vi "干啮合测试.vi"(8 "error in (no error)":errorcluster caption="错误输入（无错误）") -> (0 "error out":errorcluster caption="错误输出")   [LabVIEW 2015]
doc: "该连续测量范例项目在队列消息处理器模板的基础上实现。\n\n事件处理循环负责按用户界面操作生成对应的消息。\n\n消息处理循环负责对事件处理循环或其他消息生成的消息进行处理。其中还包括用于采集和记录消息处理循环的子VI，以及用于更新图表的循环。"
uses:
  Settings/Settings.ctl
  Acquisition/Hardware Configuration.ctl
  Logging/Logging Configuration.ctl
  Motor Control/Hardware Configuration.ctl
  controls/UI Data.ctl
  controls/UI State.ctl
  Measure Type.ctl
  <vilib>/Analysis/baseanly.llb/Mean (DBL).vi
  support/Message Queue/Enqueue Message (Single).vi
  <vilib>/Utility/error.llb/Error Cluster From Error Code.vi
  <vilib>/ErrorRing/Error Ring.xnode
  Acquisition/Acquisition.lvlib
  Logging/Logging.lvlib
  Settings/Settings.lvlib
  support/User Event - Stop/User Event - Stop.lvlib
  support/Message Queue/Message Queue.lvlib
  Motor Control/Motor Control.lvlib
  <vilib>/Analysis/NI_AALBase.lvlib
panel:
  out "XY Graph":cluster{"Y":dbl[], "Y":dbl[]}[](graph) caption="角度VS扭矩图"
  in  "设置":bool
  in  "清零":bool
  in  "读取":bool
  out "模拟通道5":dbl
  out "流量":dbl
  out "右推力":dbl
  out "左推力":dbl
  out "油压":dbl
  out "扭矩":dbl
  out "角度":dbl
  in  "计算":bool
  in  "Start":bool caption="开始"
  in  "Stop":bool caption="停止"
  out "Status":string caption="状态"
  in  "Exit":bool caption="退出"
  # "干啮合测试"
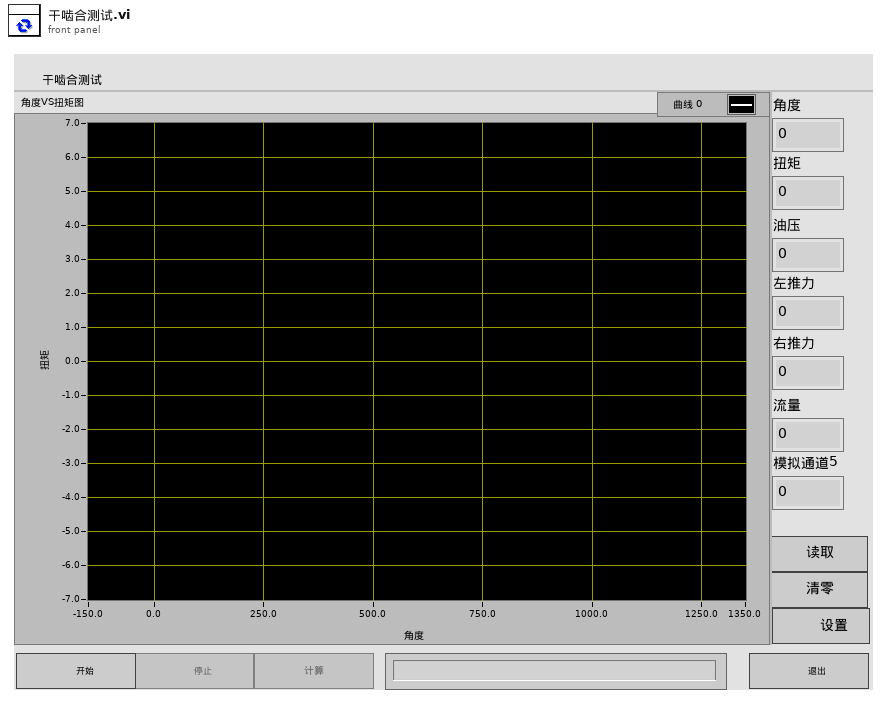
[diagram p1: front panel]
types:
  T1 = typedef "Motor Control.lvlib/电机转动逻辑1.ctl" = cluster{"反转判断条件1":T2, "停止判断条件1":T3}
  T2 = typedef "Motor Control.lvlib/反转判断条件1.ctl" = cluster{"传感器序号":i32, "条件":enum16{"小于", "大于", "等于"}, "值":dbl, "条件判断时间间隔":i32}
  T3 = typedef "Motor Control.lvlib/停止判断条件1.ctl" = cluster{"角度传感器序号":i32, "正转/反转":enum16{"正转", "反转"}, "反转次数":i32, "停止角度":dbl, "停止角度误差范围":dbl}
  T4 = typedef "UI State.ctl" = enum16{"Idle", "Acquiring and Logging", "Waiting for Exit", "Waiting for Exit (Acq Stopped)", "Waiting for Exit (Log Stopped)", "Waiting for Stop", "Waiting for Stop (Acq Stopped)", "Waiting for Stop (Log Stopped)"}
  T5 = typedef "UI Data.ctl" = cluster{"Start Ref":refnum<vi>, "Stop Ref":refnum<vi>, "calculate Ref":refnum<vi>, "Status Ref":refnum<vi>, "Exit Ref":refnum<vi>, "read Ref":refnum<vi>, "clean Ref":refnum<vi>}
  T6 = typedef "Settings.lvlib/Settings.ctl" = cluster{"Hardware Configuration":T7, "Logging Configuration":T8, "电机设置":T9, "啮合测试电机转动逻辑":T1, "功能测试电机转动逻辑":T1, "力提特性电机转动逻辑":T1}
  T7 = typedef "Acquisition.lvlib/Hardware Configuration.ctl" = cluster{"电压读取设置":cluster{"DAQmx Channel":tag, "Max Input":dbl, "Min Input":dbl, "Sample Rate":dbl, "Sample Number":i32, "DAQmx Task":refnum<k21>, "device in":tag}, "角度传感器设置":cluster{"counter":tag, "units":i32, "分辨率":i32, "初始角度":dbl, "DecodingType":i32, "A相端口":tag, "B相端口":tag, "task in":refnum<k21>}}
  T8 = typedef "Logging.lvlib/Logging Configuration.ctl" = cluster{"Log File Base Path":path, "电压传感器转换率":dbl[], "电压传感器本底":dbl[]}
  T9 = typedef "Motor Control.lvlib/Hardware Configuration.ctl" = cluster{"counter":tag, "方向端口":tag, "当前方向":bool, "频率":dbl, "DAQmx Task":refnum<k21>}
  T10 = typedef "Message Queue.lvlib/All Message Queues.ctl" = cluster{"UI":refnum<queue>, "Acquisition":refnum<queue>, "Logging":refnum<queue>, "MotorCtrl":refnum<queue>, "plot logic":refnum<queue>}
  T11 = typedef "Measure Type.ctl" = enum16{"啮合", "退回", "功能", "力特性"}
  T12 = enum8{"Enabled", "Disabled", "Disabled and Grayed Out"}
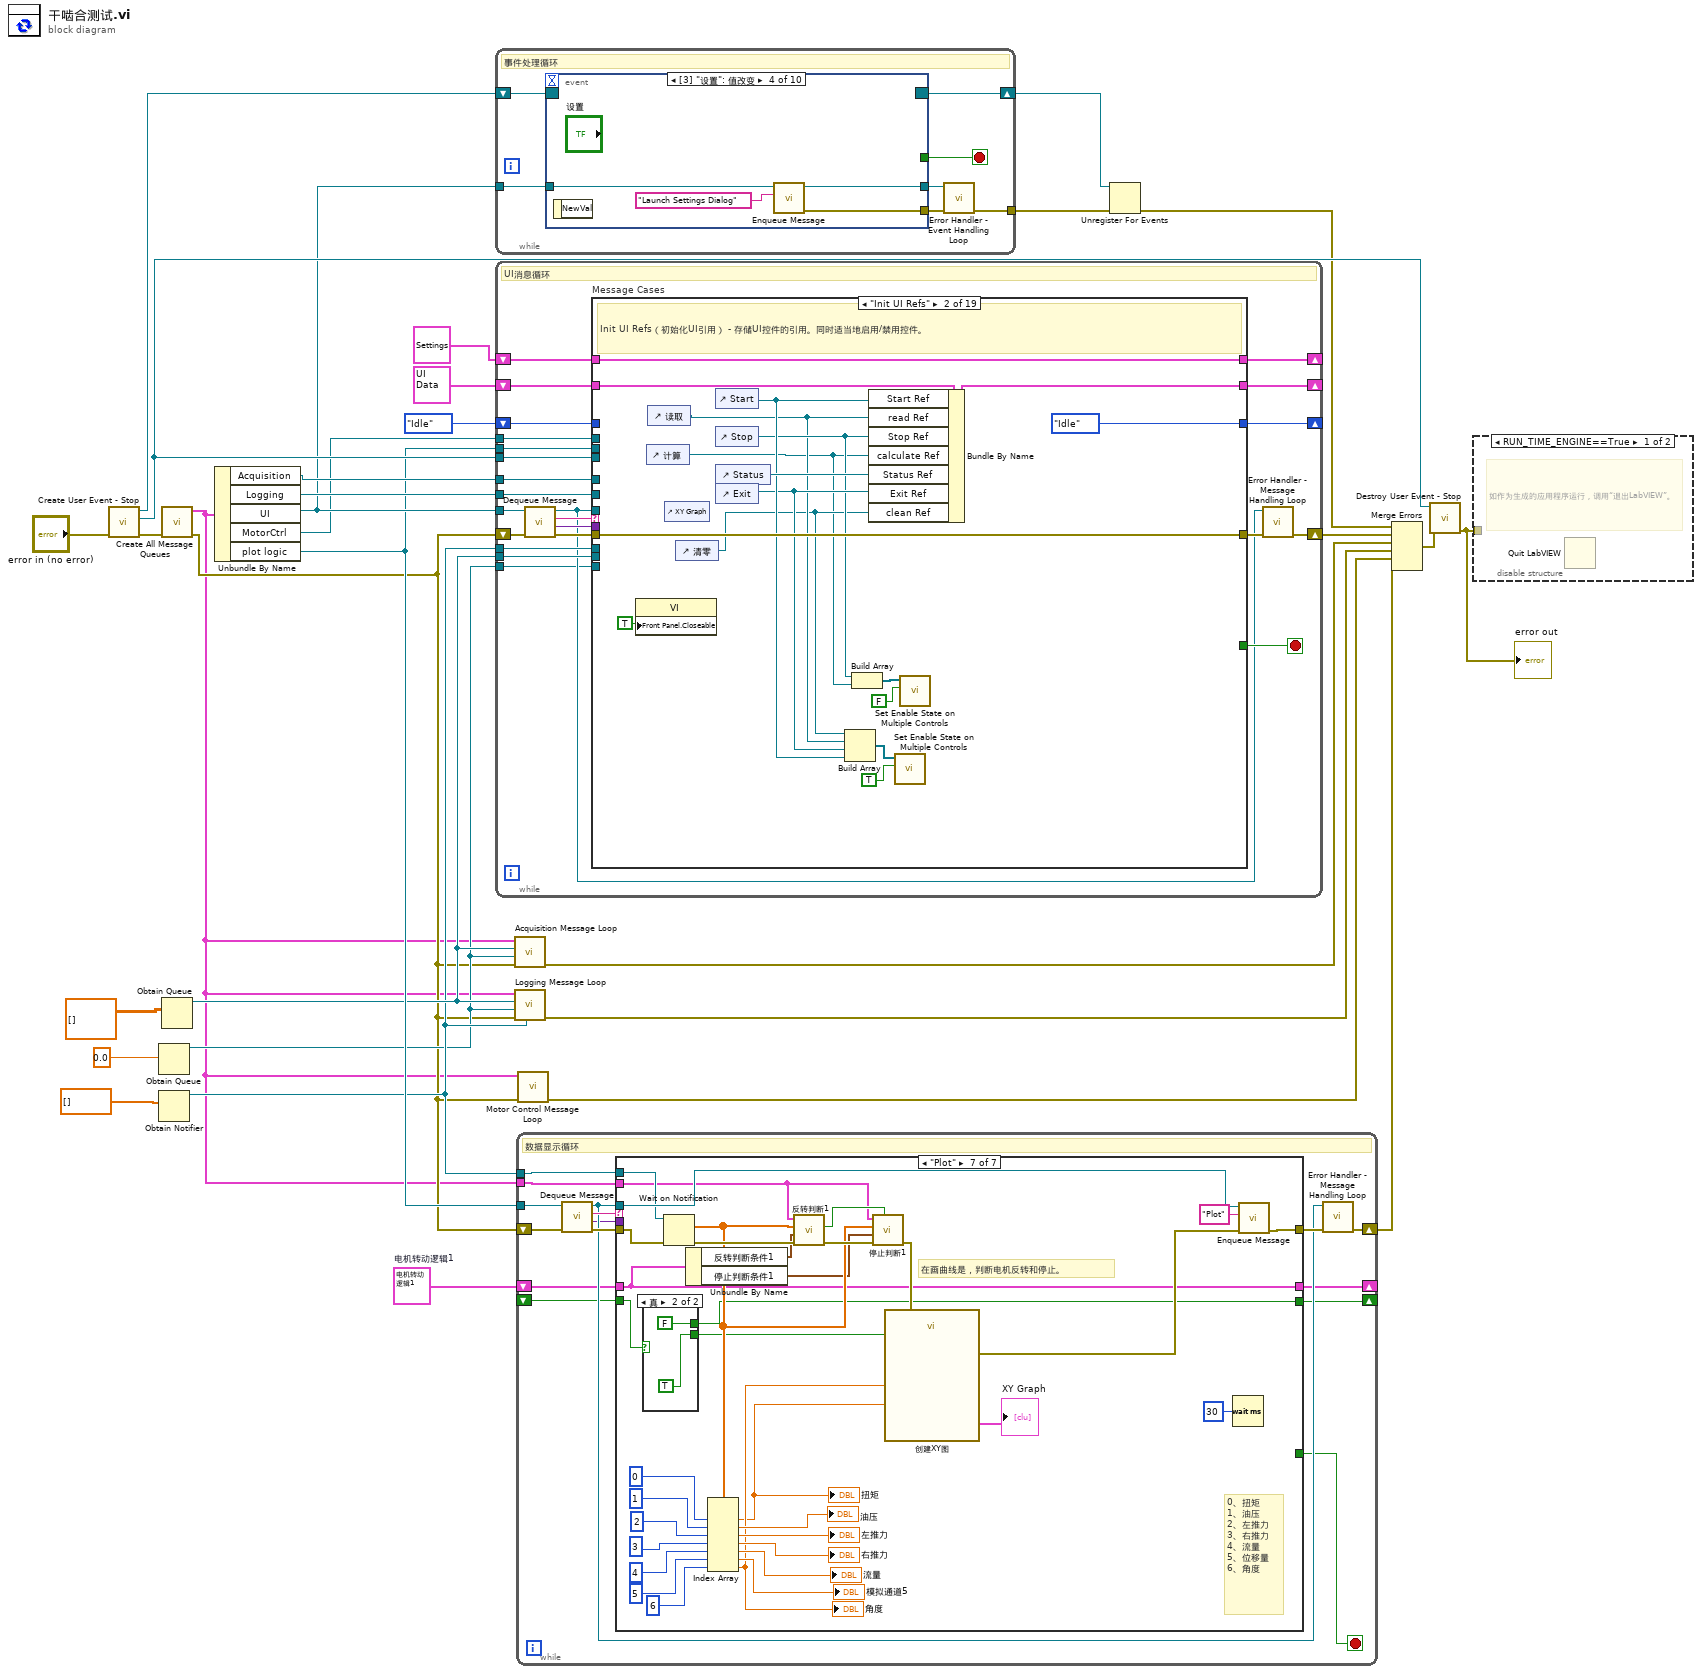
[diagram p0: block diagram]
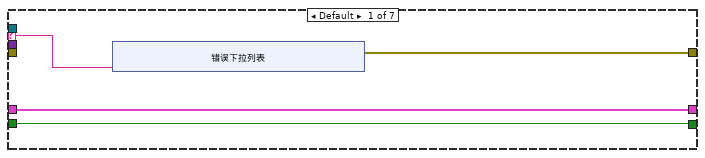
[diagram p3: hidden frame]
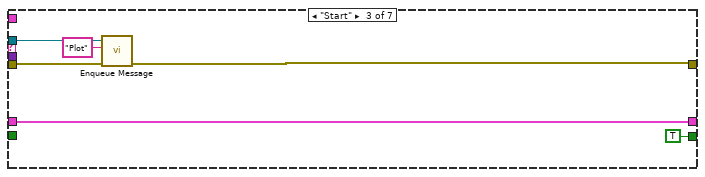
[diagram p5: hidden frame]
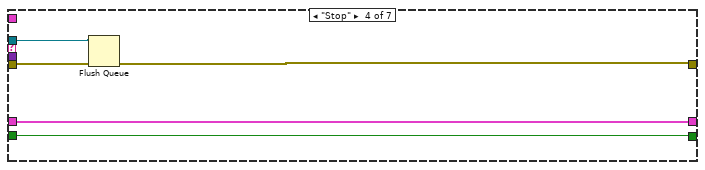
[diagram p6: hidden frame]
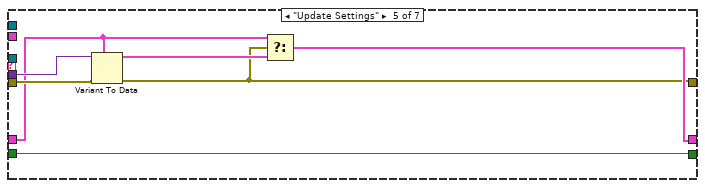
[diagram p7: hidden frame]
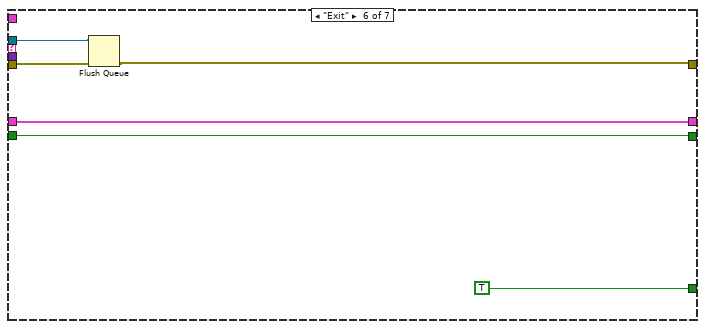
[diagram p8: hidden frame]
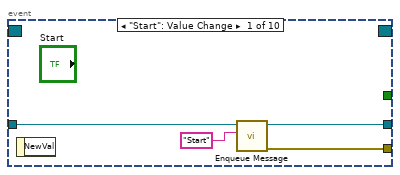
[diagram p10: hidden frame]
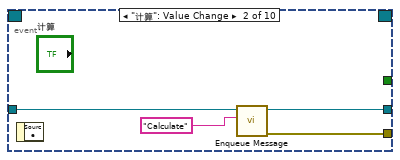
[diagram p11: hidden frame]
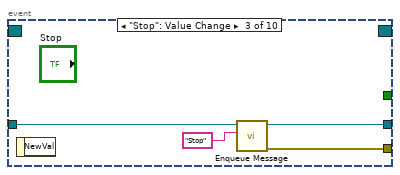
[diagram p12: hidden frame]
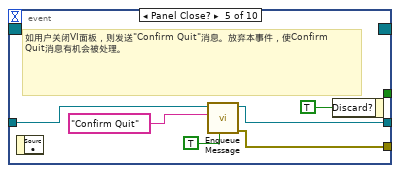
[diagram p13: hidden frame]
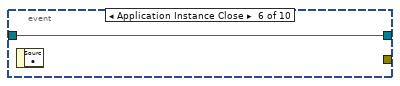
[diagram p14: hidden frame]
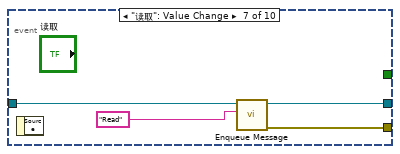
[diagram p15: hidden frame]
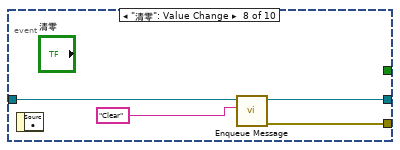
[diagram p16: hidden frame]
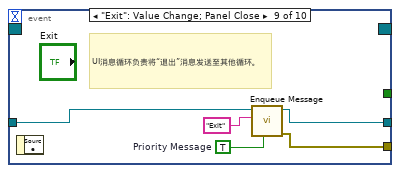
[diagram p17: hidden frame]
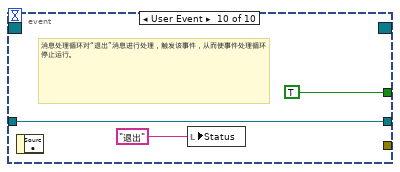
[diagram p18: hidden frame]
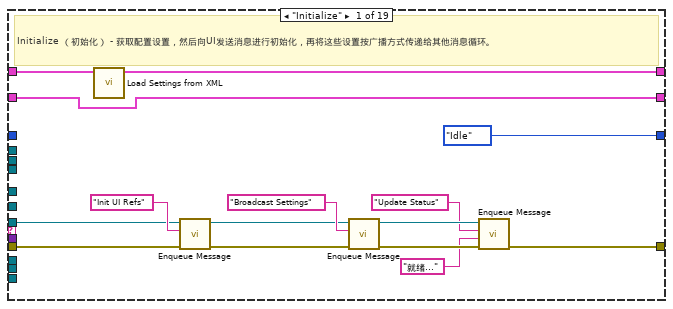
[diagram p19: hidden frame]
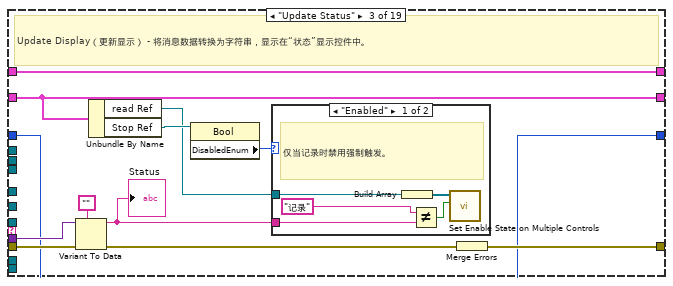
[diagram p20: hidden frame]
diagram:
  w3 = T1 {"反转判断条件1"={"传感器序号"=0, "条件"=enum."小于", "值"=0.0, "条件判断时间间隔"=0}, "停止判断条件1"={"角度传感器序号"=0, "正转/反转"=enum."正转", "反转次数"=0, "停止角度"=0.0, "停止角度误差范围"=0.0}}  # 电机转动逻辑1
  n1 = call "Create User Event - Stop.vi"("error in (no error)"="error in (no error)") -> ("error out"=w25:errorcluster, "User Event - Stop"=w27:refnum<user-event>, "Stop Event Registration Refnum"=w28:refnum<event-registration>)  [unwired: 8 in]
  n2 = Obtain Queue(element data type=0.0) -> (queue out=w8:refnum<queue>)  [unwired: 4 in, 2 out]
  n3 = Obtain Notifier(notification data type=dbl[] []) -> (notifier out=w10:refnum<notifier>)  [unwired: 3 in, 2 out]
  n4 = call "Create All Message Queues.vi"("error in (no error)"=w25) -> ("error out"=w7:errorcluster, "Message Queues out"=w4:T10)  [unwired: 9 in]
  n5 = Obtain Queue(element data type=dbl[][] []) -> (queue out=w11:refnum<queue>)  [unwired: 4 in, 2 out]
  n6 = Unbundle By Name(w4) -> ("Acquisition"=w19:refnum<queue>, "Logging"=w18:refnum<queue>, "UI"=w17:refnum<queue>, "MotorCtrl"=w15:refnum<queue>, "plot logic"=w14:refnum<queue>)
  n7 = while {
    tunnel: w17 -> [w37]
    tunnel: [w32] -> w30
    shift-right: [w36] -> w21
    shift-left: w28 -> [w38]
    stop <- w35 stop-if-true
    # "事件处理循环"
    n8 = event shown="[3] \"设置\": 值改变" {
      selector: w38 -> [_ _ _ _ _ _ _ _ _ _]
      dyn-events: [_ _ _ _ _ _ _ _ _ _] -> w36
      timeout: _ -> [_ _ _ _ _ _ _ _ _ _]
      tunnel: [_ _ _ _ _ _ _ _ _ TRUE ("Discard?")] -> w35
      tunnel: w37 -> [w40 w45 w49 w53 w60 w61 w63 w67 w71 w75]
      tunnel: [w42 w44 w48 w52 w55 _ w65 w69 w74 _] -> w33
      tunnel: [w39 w43 w47 w51 w56 w61 w62 w66 w70 w75] -> w34
      event "Start": Value Change {
        n9 = event-data() -> ()  [unwired: 1 in, 1 out]
        n10 = call-poly "Enqueue Message.vi"("Message"="Start", "Message Queue"=w40) -> ("error out"=w42:errorcluster, "dup Message Queue"=w39:refnum<queue>)  [unwired: 8 in]
      }
      event "计算": Value Change {
        n11 = event-data() -> ()  [unwired: 1 in, 1 out]
        n12 = call-poly "Enqueue Message.vi"("Message"="Calculate", "Message Queue"=w45) -> ("error out"=w44:errorcluster, "dup Message Queue"=w43:refnum<queue>)  [unwired: 8 in]
      }
      event "Stop": Value Change {
        n13 = event-data() -> ()  [unwired: 1 in, 1 out]
        n14 = call-poly "Enqueue Message.vi"("Message"="Stop", "Message Queue"=w49) -> ("error out"=w48:errorcluster, "dup Message Queue"=w47:refnum<queue>)  [unwired: 8 in]
      }
      event "设置": Value Change {
        n15 = event-data() -> ()  [unwired: 1 in, 1 out]
        n16 = call-poly "Enqueue Message.vi"("Message"="Launch Settings Dialog", "Message Queue"=w53) -> ("error out"=w52:errorcluster, "dup Message Queue"=w51:refnum<queue>)  [unwired: 8 in]
      }
      event Panel Close? {
        # "如用户关闭VI面板，则发送\"Confirm Quit\"消息。放弃本事件，使Confirm Quit消息有机会被处理。"
        n17 = event-data() -> ()  [unwired: 1 in, 1 out]
        n18 = call-poly "Enqueue Message.vi"("Priority Message? (F)"=TRUE, "Message"="Confirm Quit", "Message Queue"=w60) -> ("error out"=w55:errorcluster, "dup Message Queue"=w56:refnum<queue>)  [unwired: 7 in]
        n19 = event-data("Discard?"=TRUE) -> ()  [unwired: 1 in, 1 out]
      }
      event Application Instance Close {
        n20 = event-data() -> ()  [unwired: 1 in, 1 out]
      }
      event "读取": Value Change {
        n21 = event-data() -> ()  [unwired: 1 in, 1 out]
        n22 = call-poly "Enqueue Message.vi"("Message"="Read", "Message Queue"=w63) -> ("error out"=w65:errorcluster, "dup Message Queue"=w62:refnum<queue>)  [unwired: 8 in]
      }
      event "清零": Value Change {
        n23 = event-data() -> ()  [unwired: 1 in, 1 out]
        n24 = call-poly "Enqueue Message.vi"("Message"="Clear", "Message Queue"=w67) -> ("error out"=w69:errorcluster, "dup Message Queue"=w66:refnum<queue>)  [unwired: 8 in]
      }
      event "Exit": Value Change; Panel Close {
        w72 = TRUE  # Priority Message
        # "UI消息循环负责将“退出”消息发送至其他循环。"
        n25 = event-data() -> ()  [unwired: 1 in, 1 out]
        n26 = call-poly "Enqueue Message.vi"("Priority Message? (F)"=w72, "Message"="Exit", "Message Queue"=w71) -> ("error out"=w74:errorcluster, "dup Message Queue"=w70:refnum<queue>)  [unwired: 7 in]
      }
      event User Event {
        # "消息处理循环对“退出”消息进行处理，触发该事件，从而使事件处理循环停止运行。"
        n27 = event-data() -> ()  [unwired: 1 in, 1 out]
        n28 = local write "Status"("退出" ("Exit String")) -> ()
      }
    }
    n29 = call "Error Handler - Event Handling Loop.vi"("error in (no error)"=w33, "Message Queue"=w34) -> ("dup error in"=w32:errorcluster)  [unwired: 8 in, 1 out]
  }
  n30 = while {
    tunnel: w17 -> [w94]
    tunnel: w27 -> [w99]
    shift-right: [w84] -> w31
    shift-left: w7 -> [w98]
    shift-right: [w93] -> _
    shift-left: T6 {"Hardware Configuration"={"电压读取设置"={"DAQmx Channel"="", "Max Input"=0.0, "Min Input"=0.0, "Sample Rate"=0.0, "Sample Number"=0, "DAQmx Task"="", "device in"=""}, "角度传感器设置"={"counter"="Dev1/ctr0", "units"=10146, "分辨率"=0, "初始角度"=0.0, "DecodingType"=10092, "A相端口"="/Dev1/PFI8", "B相端口"="/Dev1/PFI8", "task in"=""}}, "Logging Configuration"={"Log File Base Path"=path "", "电压传感器转换率"=[], "电压传感器本底"=[]}, "电机设置"={"counter"="Dev1/ctr0", "方向端口"="", "当前方向"=FALSE, "频率"=0.0, "DAQmx Task"=""}, "啮合测试电机转动逻辑"={"反转判断条件1"={"传感器序号"=0, "条件"=enum."小于", "值"=0.0, "条件判断时间间隔"=0}, "停止判断条件1"={"角度传感器序号"=0, "正转/反转"=enum."正转", "反转次数"=0, "停止角度"=0.0, "停止角度误差范围"=0.0}}, "功能测试电机转动逻辑"={"反转判断条件1"={"传感器序号"=0, "条件"=enum."小于", "值"=0.0, "条件判断时间间隔"=0}, "停止判断条件1"={"角度传感器序号"=0, "正转/反转"=enum."正转", "反转次数"=0, "停止角度"=0.0, "停止角度误差范围"=0.0}}, "力提特性电机转动逻辑"={"反转判断条件1"={"传感器序号"=0, "条件"=enum."小于", "值"=0.0, "条件判断时间间隔"=0}, "停止判断条件1"={"角度传感器序号"=0, "正转/反转"=enum."正转", "反转次数"=0, "停止角度"=0.0, "停止角度误差范围"=0.0}}} ("Settings") -> [w92]
    shift-right: [w90] -> _
    shift-left: T5 {"Start Ref"=refnum, "Stop Ref"=refnum, "calculate Ref"=refnum, "Status Ref"=refnum, "Exit Ref"=refnum, "read Ref"=refnum, "clean Ref"=refnum} ("Measurement UI Controls") -> [w91]
    tunnel: w19 -> [w89]
    tunnel: w18 -> [w88]
    tunnel: w10 -> [w87]
    tunnel: w11 -> [w86]
    shift-right: [w81] -> _
    shift-left: UI_State."Idle" ("UI State") -> [w82]
    tunnel: w15 -> [w78]
    tunnel: w14 -> [w79]
    tunnel: w8 -> [w80]
    stop <- w100 stop-if-true
    # "UI消息循环"
    n31 = call "Dequeue Message.vi"("error in (no error)"=w98, "Message Queue"=w94) -> ("error out"=w97:errorcluster, "Message Data"=w95:variant, "Message"=w96:string, "dup Message Queue"=w83:refnum<queue>)  [unwired: 6 in]
    n32 = case "Message Cases" shown="\"Init UI Refs\"" w96 {
      selector: w96 -> [_ _ _ _ _ _ _ _ _ _ _ _ _ _ _ _ _ _ w430]
      tunnel: w83 -> [w105 _ _ w179 _ w219 w223 w248 _ w296 w317 w323 w361 _ _ w389 _ _ _]
      tunnel: w97 -> [w104 w132 w143 w178 w185 w218 w225 w250 w273 w298 w310 w322 w368 w375 w379 w392 w416 w424 _]
      tunnel: [w111 w132 w144 w180 w188 w220 w224 w249 w290 w293 w313 w321 w369 w374 w382 w395 w419 w428 w431] -> w85
      tunnel: [_ _ _ _ _ _ _ _ _ _ _ _ TRUE _ _ _ _ _ _] -> w100
      tunnel: w95 -> [_ _ w142 _ _ _ _ _ _ _ w309 _ _ _ _ _ _ _ _]
      tunnel: w99 -> [_ _ _ _ _ _ _ _ _ _ _ _ w367 _ _ _ _ _ _]
      tunnel: [w114 w131 w139 w177 w187 w217 w229 w254 w288 w295 w319 w326 w365 w373 w377 w385 w401 w427 w433] -> w93
      tunnel: w92 -> [w115 w131 w139 w177 w187 w217 w229 w254 w288 w299 w319 w326 w365 w373 w377 w386 w401 w427 w433]
      tunnel: w91 -> [w107 w130 w138 w174 w186 w214 w228 w253 w285 w292 w318 w325 w364 w372 w381 w394 w418 w426 w432]
      tunnel: [w107 w129 w138 w174 w186 w214 w228 w253 w285 w292 w318 w325 w364 w372 w381 w394 w418 w426 w432] -> w90
      tunnel: w89 -> [_ _ _ w162 _ w202 _ _ w284 _ _ _ w363 _ _ _ _ _ _]
      tunnel: w88 -> [_ _ _ w164 w182 w205 _ _ w283 _ _ _ w362 _ _ _ _ w422 _]
      tunnel: w87 -> [_ _ _ _ _ _ _ _ _ _ _ _ w360 _ _ _ _ _ _]
      tunnel: w86 -> [_ _ _ _ _ _ _ _ _ _ _ _ w357 _ _ _ _ _ _]
      tunnel: w82 -> [_ _ w133 _ w181 w200 w227 w252 w282 w291 w312 w324 _ w371 w380 w393 w417 w425 w429]
      tunnel: [UI_State."Idle" ("UI State") UI_State."Idle" ("UI State") w133 UI_State."Acquiring and Logging" ("UI State") w181 w199 w226 w251 w282 w291 w312 w320 UI_State."Idle" ("UI State") w371 w380 w393 w417 w425 w429] -> w81
      tunnel: w80 -> [_ _ _ _ _ _ _ _ _ _ _ _ w352 _ _ _ _ _ _]
      tunnel: w79 -> [_ _ _ w156 _ w192 _ _ w277 _ _ _ w351 _ _ _ _ _ _]
      tunnel: w78 -> [_ _ _ w152 _ w190 _ _ w280 _ _ _ w350 _ _ _ _ _ _]
      frame "Initialize" {
        # "Initialize （初始化） - 获取配置设置，然后向UI发送消息进行初始化，再将这些设置按广播方式传递给其他消息循环。"
        n33 = call "Load Settings from XML.vi"("Settings in"=w115) -> ("Settings out"=w114:T6)  [unwired: 9 in, 1 out]
        n34 = call-poly "Enqueue Message.vi"("error in (no error)"=w104, "Message"="Init UI Refs", "Message Queue"=w105) -> ("error out"=w102:errorcluster, "dup Message Queue"=w103:refnum<queue>)  [unwired: 7 in]
        n35 = call-poly "Enqueue Message.vi"("error in (no error)"=w102, "Message"="Broadcast Settings", "Message Queue"=w103) -> ("error out"=w113:errorcluster, "dup Message Queue"=w112:refnum<queue>)  [unwired: 7 in]
        n36 = call-poly "Enqueue Message.vi"("error in (no error)"=w113, "Message Data"="就绪..." ("Ready..."), "Message"="Update Status", "Message Queue"=w112) -> ("error out"=w111:errorcluster)  [unwired: 6 in, 1 out]
      }
      frame "Init UI Refs" {
        # "Init UI Refs（初始化UI引用） - 存储UI控件的引用。同时适当地启用/禁用控件。"
        n37 = property class="VI"("Front Panel.Closeable"=TRUE ("Front Panel Window:Closeable")) -> ()  [unwired: 2 in, 2 out]
        n38 = control-ref of="计算"() -> (w116:refnum<vi>)
        n39 = control-ref of="读取"() -> (w118:refnum<vi>)
        n40 = control-ref of="XY Graph"() -> ()  [unwired: 1 out]
        n41 = control-ref of="清零"() -> (w117:refnum<vi>)
        n42 = control-ref of="Start"() -> (w125:refnum<vi>)
        n43 = control-ref of="Stop"() -> (w121:refnum<vi>)
        n44 = control-ref of="Status"() -> (w126:refnum<vi>)
        n45 = control-ref of="Exit"() -> (w122:refnum<vi>)
        n46 = Build Array(w117, w118, w122, w125) -> (w124:refnum<vi>[])
        n47 = Build Array(w121, w116) -> (w120:refnum<vi>[])
        n48 = Bundle By Name(cluster=w130, "Start Ref"=w125, "read Ref"=w118, "Stop Ref"=w121, "calculate Ref"=w116, "Status Ref"=w126, "Exit Ref"=w122, "clean Ref"=w117) -> (w129:T5)
        n49 = call "Set Enable State on Multiple Controls.vi"("Enable?"=TRUE, "Controls"=w124) -> ()  [unwired: 10 in]
        n50 = call "Set Enable State on Multiple Controls.vi"("Enable?"=FALSE, "Controls"=w120) -> ()  [unwired: 10 in]
      }
      frame "Update Status" {
        # "Update Display（更新显示） - 将消息数据转换为字符串，显示在“状态”显示控件中。"
        n51 = Variant To Data(error in=w143, type="", Variant=w142) -> (data=w135:string, error out=w140:errorcluster)
        "Status" <- w135
        n52 = Unbundle By Name(w138) -> ("read Ref"=w134:refnum<vi>, "Stop Ref"=w137:refnum<vi>)
        n53 = property class="Bool"(reference=w137) -> ("DisabledEnum"=w136:T12)  [unwired: 1 in, 2 out]
        n54 = case shown="\"Enabled\"" w136 {
          tunnel: w135 -> [w147 _]
          tunnel: w134 -> [w148 _]
          frame "Enabled" {
            # "仅当记录时禁用强制触发。"
            n55 = Build Array(w148) -> (w149:refnum<vi>[])
            n56 = Not Equal?(x="记录" ("Logging"), y=w147) -> (x != y?=w145:bool)
            n57 = call "Set Enable State on Multiple Controls.vi"("Enable?"=w145, "Controls"=w149) -> ()  [unwired: 10 in]
          }
          frame "Disabled", Default {
          }
        }
        n58 = Merge Errors(w140) -> (w144:errorcluster)
      }
      frame "Start" {
        # "启用：停止\n禁用：开始、退出、设置"
        # "Start（开始） - 对于已经开始的采集，启用/禁用各个按钮并更新状态显示。"
        n59 = Unbundle By Name(w174) -> ("Stop Ref"=w157:refnum<vi>, "clean Ref"=w158:refnum<vi>, "read Ref"=w159:refnum<vi>, "Start Ref"=w169:refnum<vi>, "Exit Ref"=w168:refnum<vi>, "calculate Ref"=w167:refnum<vi>)
        n60 = call-poly "Enqueue Message.vi"("error in (no error)"=w178, "Message Data"="开始" ("Waiting for trigger"), "Message"="Update Status", "Message Queue"=w179) -> ("error out"=w166:errorcluster)  [unwired: 6 in, 1 out]
        n61 = Build Array(w157) -> (w171:refnum<vi>[])
        n62 = Build Array(w158, w159, w169, w168, w167) -> (w172:refnum<vi>[])
        n63 = call-poly "Enqueue Message.vi"("error in (no error)"=w166, "Message"="Start", "Message Queue"=w164) -> ("error out"=w163:errorcluster)  [unwired: 7 in, 1 out]
        n64 = call "Set Enable State on Multiple Controls.vi"("Enable?"=TRUE, "Controls"=w171) -> ()  [unwired: 10 in]
        n65 = call "Set Enable State on Multiple Controls.vi"("Enable?"=FALSE, "Controls"=w172) -> ()  [unwired: 10 in]
        n66 = call-poly "Enqueue Message.vi"("error in (no error)"=w163, "Message"="Start", "Message Queue"=w162) -> ("error out"=w154:errorcluster)  [unwired: 7 in, 1 out]
        n67 = call-poly "Enqueue Message.vi"("error in (no error)"=w154, "Message"="Start", "Message Queue"=w156) -> ("error out"=w153:errorcluster)  [unwired: 7 in, 1 out]
        n68 = call-poly "Enqueue Message.vi"("error in (no error)"=w153, "Message"="Start", "Message Queue"=w152) -> ("error out"=w150:errorcluster)  [unwired: 7 in, 1 out]
        n69 = Merge Errors(w150) -> (w180:errorcluster)
      }
      frame "Force Trigger" {
        # "Force Trigger（强制触发） - 发送消息至记录消息循环，开始记录。"
        n70 = call-poly "Enqueue Message.vi"("error in (no error)"=w185, "Message"="Force Trigger", "Message Queue"=w182) -> ("error out"=w184:errorcluster)  [unwired: 7 in, 1 out]
        n71 = Merge Errors(w184) -> (w188:errorcluster)
      }
      frame "Stop" {
        # "停止画图、电机、记录，最后停止采集。"
        # "启用：开始、退出、设置\n禁用：停止"
        # "停止－对于已经停止的采集，启用/禁用各个按钮并更新状态显示。"
        n72 = Unbundle By Name(w214) -> ("Stop Ref"=w196:refnum<vi>, "read Ref"=w197:refnum<vi>, "clean Ref"=w198:refnum<vi>, "Start Ref"=w209:refnum<vi>, "Exit Ref"=w208:refnum<vi>, "calculate Ref"=w207:refnum<vi>)
        n73 = call-poly "Enqueue Message.vi"("error in (no error)"=w218, "Message Data"="就绪..." ("Ready..."), "Message"="Update Status", "Message Queue"=w219) -> ("error out"=w195:errorcluster)  [unwired: 6 in, 1 out]
        n74 = Build Array(w197, w198, w209, w208, w207) -> (w212:refnum<vi>[])
        n75 = Build Array(w196) -> (w211:refnum<vi>[])
        n76 = call "Set Enable State on Multiple Controls.vi"("Enable?"=TRUE, "Controls"=w212) -> ()  [unwired: 10 in]
        n77 = call "Set Enable State on Multiple Controls.vi"("Enable?"=FALSE, "Controls"=w211) -> ()  [unwired: 10 in]
        n78 = call-poly "Enqueue Message.vi"("error in (no error)"=w195, "Message"="Stop", "Message Queue"=w192) -> ("error out"=w194:errorcluster)  [unwired: 7 in, 1 out]
        n79 = call-poly "Enqueue Message.vi"("error in (no error)"=w194, "Message"="Stop", "Message Queue"=w190) -> ("error out"=w193:errorcluster)  [unwired: 7 in, 1 out]
        n80 = call-poly "Enqueue Message.vi"("error in (no error)"=w193, "Message"="Stop", "Message Queue"=w205) -> ("error out"=w204:errorcluster)  [unwired: 7 in, 1 out]
        n81 = case shown="默认" w200 {
          selector: w200 -> [_ w222]
          tunnel: [UI_State."Waiting for Stop" ("UI State") w222] -> w199
          frame Default {
          }
          frame "Waiting for Exit" {
          }
        }
        n82 = call-poly "Enqueue Message.vi"("error in (no error)"=w204, "Message"="Stop", "Message Queue"=w202) -> ("error out"=w203:errorcluster)  [unwired: 7 in, 1 out]
        n83 = Merge Errors(w203) -> (w220:errorcluster)
      }
      frame "Acquisition Stopped" {
        # "此处代码用于确定采集停止时采取何种操作。"
        n84 = case shown="\"Waiting for Stop (Log Stopped)\"" w227 {
          selector: w227 -> [w231 _ _ _ _]
          tunnel: [w231 UI_State."Waiting for Exit (Acq Stopped)" ("UI State") UI_State."Waiting for Stop (Acq Stopped)" ("UI State") UI_State."Idle" ("UI State") UI_State."Idle" ("UI State")] -> w226
          tunnel: w225 -> [w230 w232 w234 w240 w246]
          tunnel: [w230 w232 w234 w239 w245] -> w224
          tunnel: w223 -> [_ _ _ w238 w244]
          frame Default {
          }
          frame "Waiting for Exit", "Waiting for Exit (Acq Stopped)" {
          }
          frame "Waiting for Stop", "Waiting for Stop (Acq Stopped)" {
          }
          frame "Waiting for Exit (Log Stopped)" {
            # "如果正在等待退出且记录已结束，“采集停止”消息表示应退出。"
            n85 = call-poly "Enqueue Message.vi"("Priority Message? (F)"=TRUE, "error in (no error)"=w240, "Message"="Exit", "Message Queue"=w238) -> ("error out"=w239:errorcluster)  [unwired: 6 in, 1 out]
          }
          frame "Waiting for Stop (Log Stopped)" {
            # "当前状态为等待停止时，如已停止记录，则收到\"Acquisition Stopped\"消息时即可停止。"
            n86 = call-poly "Enqueue Message.vi"("error in (no error)"=w246, "Message Data"="Ready..." ("Message"), "Message"="Update Status", "Message Queue"=w244) -> ("error out"=w245:errorcluster)  [unwired: 6 in, 1 out]
          }
        }
      }
      frame "Logging Stopped" {
        # "此处代码用于确定记录停止时采取何种操作。"
        n87 = case shown="\"Waiting for Stop (Acq Stopped)\"" w252 {
          selector: w252 -> [w256 _ _ _ _]
          tunnel: [w256 UI_State."Waiting for Exit (Log Stopped)" ("UI State") UI_State."Waiting for Stop (Log Stopped)" ("UI State") UI_State."Idle" ("UI State") UI_State."Idle" ("UI State")] -> w251
          tunnel: w250 -> [w255 w257 w259 w265 w271]
          tunnel: [w255 w257 w259 w264 w270] -> w249
          tunnel: w248 -> [_ _ _ w263 w269]
          frame Default {
          }
          frame "Waiting for Exit", "Waiting for Exit (Log Stopped)" {
          }
          frame "Waiting for Stop", "Waiting for Stop (Log Stopped)" {
          }
          frame "Waiting for Exit (Acq Stopped)" {
            # "如果正在等待退出且采集已结束，“记录停止”消息表示应退出。"
            n88 = call-poly "Enqueue Message.vi"("Priority Message? (F)"=TRUE, "error in (no error)"=w265, "Message"="Exit", "Message Queue"=w263) -> ("error out"=w264:errorcluster)  [unwired: 6 in, 1 out]
          }
          frame "Waiting for Stop (Acq Stopped)" {
            # "如果正在等待停止且采集已结束，“记录停止”消息表示应停止。"
            n89 = call-poly "Enqueue Message.vi"("error in (no error)"=w271, "Message Data"="Ready..." ("Message"), "Message"="Update Status", "Message Queue"=w269) -> ("error out"=w270:errorcluster)  [unwired: 6 in, 1 out]
          }
        }
      }
      frame "Broadcast settings" {
        w276 = "Update Settings" ("Message")
        # "向“记录和采集”消息队列发送“更新设置”消息。"
        n90 = Unbundle By Name(w288) -> ("Hardware Configuration"=w287:T7, "Logging Configuration"=w286:T8, "电机设置"=w279:T9, "啮合测试电机转动逻辑"=w275:T1)
        n91 = call-poly "Enqueue Message.vi"("error in (no error)"=w273, "Message Data"=w287, "Message"=w276, "Message Queue"=w284) -> ("error out"=w289:errorcluster)  [unwired: 6 in, 1 out]
        n92 = call-poly "Enqueue Message.vi"("error in (no error)"=w289, "Message Data"=w286, "Message"=w276, "Message Queue"=w283) -> ("error out"=w281:errorcluster)  [unwired: 6 in, 1 out]
        n93 = call-poly "Enqueue Message.vi"("error in (no error)"=w281, "Message Data"=w279, "Message"=w276, "Message Queue"=w280) -> ("error out"=w278:errorcluster)  [unwired: 6 in, 1 out]
        n94 = call-poly "Enqueue Message.vi"("error in (no error)"=w278, "Message Data"=w275, "Message"=w276, "Message Queue"=w277) -> ("error out"=w274:errorcluster)  [unwired: 6 in, 1 out]
        n95 = Merge Errors(w274, w273) -> (w290:errorcluster)
      }
      frame "Launch Settings Dialog" {
        # "用户单击“设置”按钮时，启动设置对话框。"
        n96 = call "Measure Settings Dialog.vi"("error in (no error)"=w298, "Settings in"=w299) -> ("error out"=w294:errorcluster, "Cancelled?"=w297:bool, "Settings out"=w295:T6)  [unwired: 6 in, 1 out]
        n97 = case shown="假" w297 {
          tunnel: w296 -> [w303 _]
          tunnel: w294 -> [w302 w304]
          tunnel: [w301 w304] -> w293
          frame False {
            n98 = call-poly "Enqueue Message.vi"("error in (no error)"=w302, "Message"="Broadcast Settings", "Message Queue"=w303) -> ("error out"=w301:errorcluster)  [unwired: 7 in, 1 out]
          }
          frame True {
          }
        }
      }
      frame "Error" {
        # "Error - 检查错误消息数据及其响应。该消息由应用程序各循环结束处的“错误处理”VI发送。"
        n99 = Variant To Data(error in=w310, type=errorcluster {"status"=FALSE, "code"=0, "source"=""} ("错误常量"), Variant=w309) -> (data=w307:errorcluster, error out=w306:errorcluster)
        n100 = call <vilib>:"Simple Error Handler.vi"("error in (no error)"=w306) -> ("error out"=w305:errorcluster)  [unwired: 4 in, 4 out]
        n101 = call <vilib>:"Simple Error Handler.vi"("error in (no error)"=w307) -> ("error out"=w311:errorcluster)  [unwired: 4 in, 4 out]
        n102 = call-poly "Enqueue Message.vi"("Priority Message? (F)"=TRUE, "Message"="Exit", "Message Queue"=w317) -> ("error out"=w314:errorcluster)  [unwired: 7 in, 1 out]
        n103 = Merge Errors(w314, w311, w305) -> (w313:errorcluster)
      }
      frame "Confirm Quit" {
        # "Confirm Quit - 该消息用于确认用户是否需要退出应用程序。"
        n104 = case shown="\"Acquiring and Logging\"" w324 {
          tunnel: w323 -> [w331 w337]
          tunnel: w322 -> [w330 w335]
          tunnel: [w327 w334] -> w321
          tunnel: [UI_State."Idle" ("UI State") w333] -> w320
          frame Default {
            # "如收到'Confirm Quit'消息时系统处于空闲状态，则不需要弹出确认提示。"
            n105 = call-poly "Enqueue Message.vi"("Priority Message? (F)"=TRUE, "error in (no error)"=w330, "Message"="Exit", "Message Queue"=w331) -> ("error out"=w327:errorcluster)  [unwired: 6 in, 1 out]
          }
          frame "Acquiring and Logging" {
            n106 = Two Button Dialog(message="采集仍在执行中，是否确定退出？" ("Confirm Quit Message"), 1:"否" ("No"), 2:"是" ("Yes")) -> (T button?=w336:bool)
            n107 = case shown="真" w336 {
              tunnel: w337 -> [_ w347]
              tunnel: w335 -> [w341 w346]
              tunnel: [w341 w345] -> w334
              tunnel: [UI_State."Acquiring and Logging" ("UI State") UI_State."Waiting for Exit" ("UI State")] -> w333
              frame False {
                # "用户不希望退出。"
              }
              frame True {
                n108 = call-poly "Enqueue Message.vi"("error in (no error)"=w346, "Message"="Stop", "Message Queue"=w347) -> ("error out"=w345:errorcluster)  [unwired: 7 in, 1 out]
              }
            }
          }
        }
      }
      frame "Exit" {
        w348 = TRUE ("Priority Message? (F)")
        w349 = "Exit" ("Message")
        # "不必检查错误输出。采集和记录队列可能已被释放。"
        # "停止VI。"
        # "Exit（退出）－触发用户事件，使“事件处理”循环停止运行。同时向“采集和记录”循环发送“退出”消息。"
        n109 = Release Queue(queue=w361, error in (no error)=w368) -> (error out=w359:errorcluster)  [unwired: 1 in, 2 out]
        n110 = call "Fire User Event - Stop.vi"("User Event - Stop"=w367) -> ("error out"=w366:errorcluster)  [unwired: 10 in]
        n111 = Release Notifier(notifier=w360, error in (no error)=w359) -> (error out=w358:errorcluster)  [unwired: 1 in, 2 out]
        n112 = Release Queue(queue=w357, error in (no error)=w358) -> (error out=w354:errorcluster)  [unwired: 1 in, 2 out]
        n113 = call-poly "Enqueue Message.vi"("Priority Message? (F)"=TRUE, "Message"=w349, "Message Queue"=w363) -> ()  [unwired: 7 in, 2 out]
        n114 = Release Queue(queue=w352, error in (no error)=w354) -> (error out=w353:errorcluster)  [unwired: 1 in, 2 out]
        n115 = call-poly "Enqueue Message.vi"("Priority Message? (F)"=w348, "Message"=w349, "Message Queue"=w362) -> ()  [unwired: 7 in, 2 out]
        n116 = call-poly "Enqueue Message.vi"("Priority Message? (F)"=w348, "Message"=w349, "Message Queue"=w351) -> ()  [unwired: 7 in, 2 out]
        n117 = call-poly "Enqueue Message.vi"("Priority Message? (F)"=w348, "Message"=w349, "Message Queue"=w350) -> ()  [unwired: 7 in, 2 out]
        n118 = Merge Errors(w366, w353) -> (w369:errorcluster)
      }
      frame "---Copy This Frame---" {
        # "如需创建新消息，可创建该帧的副本。在副本中，将本注释更改为对应消息的注释。"
        n119 = Merge Errors(w375) -> (w374:errorcluster)
      }
      frame "DAQ Reset" {
        # "如需创建新消息，可创建该帧的副本。在副本中，将本注释更改为对应消息的注释。"
        n120 = Unbundle By Name(w377) -> ("Hardware Configuration.电压读取设置.device in"=w376:tag)
        n121 = call <vilib>:"DAQmx Reset Device.vi"("device in"=w376, "error in"=w379) -> ("error out"=w378:errorcluster)  [unwired: 13 in]
        n122 = Merge Errors(w378) -> (w382:errorcluster)
      }
      frame "Clear" {
        # "如需创建新消息，可创建该帧的副本。在副本中，将本注释更改为对应消息的注释。"
        n123 = call "Acquire Once.vi"("error in (no error)"=w392, "Settings"=w386) -> ("error out"=w391:errorcluster, "信号数据"=w384:dbl[][])  [unwired: 7 in, 1 out]
        n124 = for {
          tunnel: w384 -> [w397] mode=indexing
          tunnel: [w396] -> w383 mode=indexing
          n125 = call-poly <vilib>:"Mean.vi"("X"=w397) -> ("mean"=w396:dbl)  [unwired: 1 out]
        }
        n126 = Bundle By Name(cluster=w386, "Logging Configuration.电压传感器本底"=w383) -> (w385:T6)
        n127 = call "Save Settings to XML.vi"("error in (no error)"=w391, "Settings"=w385) -> ("error out"=w388:errorcluster)  [unwired: 9 in]
        n128 = call-poly "Enqueue Message.vi"("error in (no error)"=w388, "Message"="Broadcast Settings", "Message Queue"=w389) -> ("error out"=w387:errorcluster)  [unwired: 7 in, 1 out]
        n129 = Merge Errors(w387) -> (w395:errorcluster)
      }
      frame "Read" {
        # "如需创建新消息，可创建该帧的副本。在副本中，将本注释更改为对应消息的注释。"
        n130 = call "Acquire Once.vi"("error in (no error)"=w416, "Settings"=w401) -> ("error out"=w415:errorcluster, "信号数据"=w402:dbl[][])  [unwired: 7 in, 1 out]
        n131 = Unbundle By Name(w401) -> ("Logging Configuration.电压传感器转换率"=w400:dbl[], "Logging Configuration.电压传感器本底"=w399:dbl[])
        n132 = call "GetDatas.vi"("电压传感器本地"=w399, "电压传感器转换率"=w400, "信号数据"=w402) -> ("传感器信号"=w398:dbl[])  [unwired: 8 in]
        n133 = Index Array(array=w398, index #1=0 ("索引"), index #2=1 ("索引"), index #3=2 ("索引"), index #4=3 ("索引"), index #5=4 ("索引"), index #6=5 ("索引")) -> (element #1=w408:dbl, element #2=w407:dbl, element #3=w406:dbl, element #4=w405:dbl, element #5=w404:dbl, element #6=w403:dbl)
        n134 = local write "扭矩"(w408) -> ()
        n135 = local write "左推力"(w406) -> ()
        n136 = local write "油压"(w407) -> ()
        n137 = local write "模拟通道5"(w403) -> ()
        n138 = local write "右推力"(w405) -> ()
        n139 = local write "流量"(w404) -> ()
        n140 = Merge Errors(w415) -> (w419:errorcluster)
      }
      frame "Calculate" {
        # "发指令让记录线程执行计算，传入相应的计算类型。"
        # "如需创建新消息，可创建该帧的副本。在副本中，将本注释更改为对应消息的注释。"
        n141 = call-poly "Enqueue Message.vi"("error in (no error)"=w424, "Message Data"=Measure_Type."啮合" ("计算类型"), "Message"="Calculate", "Message Queue"=w422) -> ("error out"=w423:errorcluster)  [unwired: 6 in, 1 out]
        n142 = Merge Errors(w423) -> (w428:errorcluster)
      }
      frame Default {
        # "如得到的消息未经任何分支定义，则运行“默认”分支。输出程序错误。"
        n143 = xnode "错误下拉列表"("参数 0"=w430) -> ("错误输出"=w431:errorcluster)
      }
    }
    n144 = call "Error Handler - Message Handling Loop.vi"("error in (no error)"=w85, "Message Queue"=w83) -> ("dup error in"=w84:errorcluster)  [unwired: 8 in, 1 out]
  }
  n145 = call "Acquisition Message Loop.vi"("error in (no error)"=w7, "Angle Data Queue"=w8, "Analog Data Queue"=w11, "Message Queues"=w4) -> ("error out"=w26:errorcluster)  [unwired: 7 in]
  n146 = call "Logging Message Loop.vi"("数据通知器"=w10, "error in (no error)"=w7, "Angle Data Queue"=w8, "Analog Data Queue"=w11, "Message Queues"=w4) -> ("error out"=w24:errorcluster)  [unwired: 6 in]
  n147 = while "Data Display Loop" {
    tunnel: w10 -> [w448]
    tunnel: w14 -> [w455]
    shift-right: [w450] -> w5
    shift-left: w7 -> [w454]
    tunnel: w4 -> [w446]
    shift-right: [w443] -> _
    shift-left: w3 -> [w444]
    shift-right: [w442] -> _
    shift-left: _ -> [w441]
    stop <- w447 stop-if-true
    # "数据显示循环"
    n148 = call "Dequeue Message.vi"("error in (no error)"=w454, "Message Queue"=w455) -> ("error out"=w452:errorcluster, "Message Data"=w445:variant, "Message"=w451:string, "dup Message Queue"=w449:refnum<queue>)  [unwired: 6 in]
    n149 = case shown="\"Plot\"" w451 {
      selector: w451 -> [w458 _ _ _ _ _ _]
      tunnel: [w459 w468 w472 w479 w482 w491 w509] -> w453
      tunnel: w452 -> [_ w468 w475 w480 w486 w493 w524]
      tunnel: w449 -> [_ _ w474 w478 _ w492 w527]
      tunnel: w448 -> [_ _ _ _ _ _ w525]
      tunnel: [_ _ _ _ _ TRUE _] -> w447
      tunnel: w446 -> [_ _ _ _ _ _ w503]
      tunnel: w445 -> [_ _ _ _ w485 _ _]
      tunnel: [w457 w469 w471 w477 w483 w489 w500] -> w443
      tunnel: w444 -> [w457 w469 w471 w477 w484 w489 w500]
      tunnel: [w456 w467 TRUE w476 w481 w488 w494] -> w442
      tunnel: w441 -> [w456 w467 _ w476 w481 w488 w496]
      frame Default {
        n150 = xnode "错误下拉列表"("参数 0"=w458) -> ("错误输出"=w459:errorcluster)
      }
      frame "Initialize" {
      }
      frame "Start" {
        n151 = call-poly "Enqueue Message.vi"("error in (no error)"=w475, "Message"="Plot", "Message Queue"=w474) -> ("error out"=w472:errorcluster)  [unwired: 7 in, 1 out]
      }
      frame "Stop" {
        n152 = Flush Queue(queue=w478, error in (no error)=w480) -> (error out=w479:errorcluster)  [unwired: 2 out]
      }
      frame "Update Settings" {
        n153 = Variant To Data(error in=w486, type=w484, Variant=w485) -> (data=w487:T1, error out=w482:errorcluster)
        n154 = Select(t=w484, s=w482, f=w487) -> (s? t:f=w483:T1)
      }
      frame "Exit" {
        n155 = Flush Queue(queue=w492, error in (no error)=w493) -> (error out=w491:errorcluster)  [unwired: 2 out]
      }
      frame "Plot" {
        # "在画曲线是，判断电机反转和停止。"
        # "0、扭矩\n1、油压\n2、左推力\n3、右推力\n4、流量\n5、位移量\n6、角度"
        n156 = case shown="真" w496 {
          tunnel: [_ TRUE] -> w495
          tunnel: [_ FALSE] -> w494
          frame False {
          }
          frame True {
          }
        }
        n157 = Wait on Notification(notifier=w525, error in (no error)=w524) -> (notification=w502:dbl[], error out=w506:errorcluster)  [unwired: 2 in, 2 out]
        n158 = Unbundle By Name(w500) -> ("反转判断条件1"=w499:T2, "停止判断条件1"=w498:T3)
        n159 = Index Array(array=w502, index #1=0 ("索引"), index #2=1 ("索引"), index #3=2 ("索引"), index #4=3 ("索引"), index #5=4 ("索引"), index #6=5 ("索引"), index #7=6 ("索引")) -> (element #1=w507:dbl, element #2=→"油压":dbl, element #3=→"左推力":dbl, element #4=→"右推力":dbl, element #5=→"流量":dbl, element #6=→"模拟通道5":dbl, element #7=w508:dbl)
        "角度" <- w508
        "扭矩" <- w507
        n160 = call "反转判断1.vi"("error in (no error)"=w506, "反转判断条件1"=w499, "传感器数据"=w502, "Message Queues"=w503) -> ("error out"=w505:errorcluster, "反转"=w504:bool)  [unwired: 6 in]
        n161 = call "停止判断1.vi"("反转？"=w504, "error in (no error)"=w505, "反转判断条件1"=w498, "传感器数据"=w502, "Message Queues"=w503) -> ("error out"=w501:errorcluster)  [unwired: 6 in]
        n162 = call "创建XY图"("error in (no error)"=w501, "Reset"=w495, "Y Input"=w507, "X Input"=w508) -> ("error out"=w510:errorcluster, "XY Graph"=→"XY Graph":cluster{"X":dbl[], "Y":dbl[]}[])  [unwired: 6 in]
        n163 = Wait (ms)(milliseconds to wait=u32 30 ("等待时间（毫秒）")) -> ()  [unwired: 1 out]
        n164 = call-poly "Enqueue Message.vi"("error in (no error)"=w510, "Message"="Plot", "Message Queue"=w527) -> ("error out"=w509:errorcluster)  [unwired: 7 in, 1 out]
      }
    }
    n165 = call "Error Handler - Message Handling Loop.vi"("error in (no error)"=w453, "Message Queue"=w449) -> ("dup error in"=w450:errorcluster)  [unwired: 8 in, 1 out]
  }
  n166 = call "Motor Control Message Loop.vi"("error in (no error)"=w7, "Message Queues"=w4) -> ("error out"=w6:errorcluster)  [unwired: 9 in]
  n167 = Unregister For Events(event registration refnum=w21, error in=w30) -> (error out=w22:errorcluster)
  n168 = Merge Errors(w22, w31, w26, w24, w6, w5) -> (w29:errorcluster)
  n169 = call "Destroy User Event - Stop.vi"("error in (no error)"=w29, "User Event - Stop"=w27) -> ("error out"=w1:errorcluster)  [unwired: 9 in]
  "error out" <- w1
  n170 = disable-structure shown="RUN_TIME_ENGINE==True" {
    disable-tunnel: w1 -> [_ _]
    frame condition #0 {
      # "如作为生成的应用程序运行，调用“退出LabVIEW”。"
      n171 = Quit LabVIEW() -> ()  [unwired: 1 in]
    }
    frame condition #1 (active) {
    }
  }
